vi "Day9-2.vi"() -> ()   [LabVIEW 2021]
panel:
  out "size":i32
  out "element":cluster{"x":i32, "y":i32}
  out "Array":string[](array[string])
  out "array":string[][](array[string])
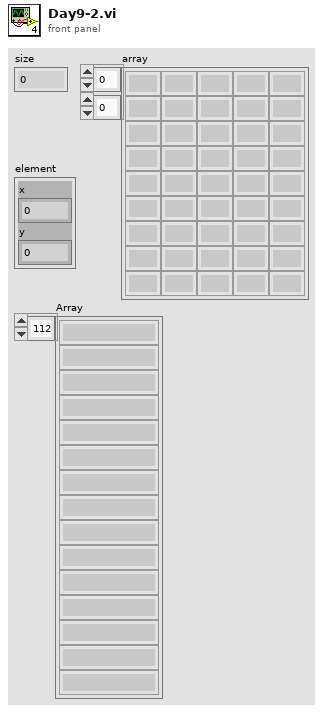
[diagram p1: front panel]
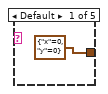
[diagram p2: hidden frame]
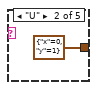
[diagram p3: hidden frame]
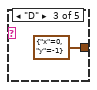
[diagram p4: hidden frame]
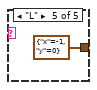
[diagram p5: hidden frame]
diagram:
  w7 = set{cluster{"x":i32, "y":i32}} {}  # Size: 0
  w11 = 10 ("dimension size")
  # "Initial starting position of Head and Tail = (0,0)"
  n1 = Spreadsheet String To Array(delimiter (Tab)=" ", format string="%s", spreadsheet string="R 2\nD 2\nR 2\nU 1\nR 2\nL 2\nD 1\nL 1\nD 2\nR 2\nU 2\nD 1\nR 2\nD 2\nU 1\nR 1\nD 1\nL 1\nU 1\nR 1\nL 1\nR 2\nU 2\nD 2\nR 2\nL 2\nU 1\nL 2\nU 2\nL 2\nR 2\nU 2\nR 1\nU 2\nL 2\nD 1\nR 1\nU 2\nD 2\nR 2\nL 2\nU 1\nD 1\nL 2\nU 2\nL 2\nU 1\nD 2\nR 1\nD 1\nR 2\nU 1\nL 2\nD 1\nU 2\nR 2\nL 1\nD 2\nU 1\nD 1\nL 1\nU 1\nR 1\nD 1\nR 1\nU 1\nD 2\nL 1\nD 1\nR 2\nD 1\nU 2\nD 2\nU 2\nL 1\nU 2\nR 2\nL 2\nD 2\nR 1\nL 2\nU 2\nL 1\nU 1\nL 1\nR 2\nL 2\nR 1\nD 1\nU 1\nL 2\nR 1\nL 1\nU 1\nD 1\nU 1\nD 1\nR 1\nL 2\nR 2\nL 1\nU 1\nD 2\nU 2\nL 2\nR 2\nU 1\nR 2\nL 2\nR 2\nL 1\nU 3\nD 1\nL 1\nD 3\nU 1\nD 2\nL 1\nR 3\nD 2\nU 3\nR 1\nD 3\nR 2\nD 1\nU 3\nL 1\nR 2\nL 3\nD 3\nU 2\nL 2\nR 3\nU 3\nD 3\nL 3\nD 2\nL 3\nR 1\nL 1\nD 1\nU 3\nD 3\nU 2\nL 3\nR 3\nU 1\nD 2\nR 2\nL 2\nD 3\nR 3\nU 1\nR 1\nL 3\nU 2\nL 2\nU 1\nR 1\nD 1\nR 3\nU 2\nD 1\nL 1\nU 1\nR 2\nL 1\nR 3\nL 1\nU 3\nL 2\nD 2\nL 2\nD 3\nL 2\nR 1\nU 2\nL 3\nD 1\nL 3\nD 1\nU 2\nL 3\nR 2\nU 1\nL 3\nD 3\nR 3\nU 2\nR 2\nD 3\nR 3\nU 2\nR 2\nL 2\nU 3\nR 1\nL 2\nD 3\nU 1\nL 1\nU 1\nL 2\nR 3\nL 3\nD 3\nR 3\nU 3\nL 1\nR 2\nD 3\nU 1\nR 2\nU 1\nD 1\nL 1\nD 2\nL 2\nD 3\nU 2\nD 1\nU 3\nD 3\nU 3\nR 3\nL 3\nU 4\nL 3\nD 1\nR 4\nU 3\nD 2\nR 1\nD 4\nL 3\nU 1\nL 1\nR 2\nD 1\nR 3\nD 3\nL 3\nD 4\nL 3\nR 4\nU 3\nR 3\nD 1\nR 3\nD 3\nR 3\nD 4\nU 4\nR 2\nD 3\nR 3\nD 2\nU 1\nR 2\nD 2\nU 2\nD 3\nL 2\nR 4\nD 4\nU 4\nR 3\nU 4\nR 1\nU 2\nR 4\nD 2\nL 4\nR 4\nU 3\nL 2\nU 2\nL 3\nR 3\nL 1\nU 4\nL 3\nU 3\nL 3\nU 1\nR 2\nU 3\nR 2\nL 3\nU 1\nD 3\nR 4\nD 1\nR 2\nL 1\nD 1\nU 2\nD 3\nR 4\nU 1\nL 3\nR 4\nU 4\nL 4\nR 2\nD 1\nU 4\nR 1\nD 3\nL 3\nD 1\nR 3\nD 2\nU 2\nL 1\nU 2\nD 3\nL 1\nU 3\nD 3\nL 3\nU 2\nL 3\nU 2\nR 1\nD 1\nR 1\nL 1\nD 2\nR 3\nD 2\nL 2\nR 3\nD 5\nR 5\nU 4\nD 5\nU 5\nD 4\nR 4\nD 2\nR 5\nL 4\nR 2\nL 2\nR 5\nU 5\nR 1\nD 2\nR 1\nL 3\nD 5\nU 3\nD 4\nR 3\nU 4\nD 1\nU 4\nL 5\nR 1\nU 4\nL 5\nU 3\nD 4\nL 2\nD 4\nU 4\nL 2\nD 1\nR 3\nD 1\nR 2\nD 4\nR 5\nL 1\nU 4\nL 4\nU 3\nL 1\nU 1\nR 4\nU 3\nL 1\nR 3\nD 5\nU 2\nR 4\nD 3\nL 2\nD 4\nR 5\nD 2\nU 3\nR 4\nD 4\nL 2\nU 4\nR 5\nL 1\nU 5\nD 1\nR 3\nL 4\nD 1\nU 3\nD 5\nR 2\nD 2\nL 5\nU 2\nD 3\nL 5\nD 5\nL 1\nR 5\nD 2\nU 3\nR 2\nL 2\nU 1\nL 5\nR 1\nL 4\nD 5\nR 5\nD 2\nU 5\nL 5\nD 1\nL 1\nD 3\nR 1\nD 2\nL 2\nR 4\nU 5\nL 2\nR 1\nU 3\nD 1\nU 1\nD 5\nR 2\nD 2\nR 3\nD 6\nU 1\nR 6\nD 4\nU 1\nR 5\nL 6\nR 2\nL 6\nU 6\nR 5\nD 2\nU 1\nD 2\nL 2\nD 5\nR 3\nU 4\nD 2\nL 1\nU 1\nD 3\nU 1\nD 1\nR 5\nU 1\nR 1\nD 3\nU 5\nL 6\nR 3\nL 6\nU 4\nD 2\nR 1\nL 6\nR 2\nD 3\nU 2\nR 2\nL 1\nD 1\nU 1\nR 4\nU 1\nR 2\nU 2\nL 2\nU 2\nD 5\nL 4\nU 6\nL 3\nD 6\nU 5\nL 6\nU 3\nR 5\nU 2\nR 4\nL 6\nD 1\nR 5\nD 4\nL 2\nR 2\nU 1\nD 2\nL 2\nU 4\nR 1\nD 2\nU 2\nR 6\nL 2\nD 5\nR 5\nL 3\nD 1\nU 1\nL 2\nD 4\nR 6\nL 5\nR 3\nU 1\nR 3\nL 1\nR 3\nU 1\nL 1\nU 4\nD 4\nU 3\nR 3\nU 1\nR 2\nD 1\nL 6\nU 2\nR 2\nD 1\nR 5\nL 2\nD 5\nL 3\nR 6\nD 2\nL 2\nD 3\nL 5\nD 7\nL 7\nD 4\nU 5\nR 7\nL 7\nD 3\nU 5\nR 6\nU 3\nL 6\nR 5\nL 4\nD 4\nR 4\nL 6\nD 6\nU 3\nD 3\nR 7\nU 1\nL 5\nU 3\nL 4\nU 3\nL 5\nD 1\nR 7\nU 3\nL 6\nD 1\nU 3\nL 2\nU 6\nL 6\nD 1\nU 1\nD 2\nL 5\nU 4\nR 5\nD 7\nU 3\nD 4\nL 1\nD 3\nR 7\nD 2\nU 4\nL 1\nD 3\nR 3\nD 6\nR 4\nU 3\nD 4\nR 6\nL 7\nU 5\nL 7\nR 3\nL 7\nD 5\nR 7\nD 4\nU 3\nR 6\nU 7\nD 2\nR 2\nL 2\nD 1\nR 3\nU 3\nD 5\nU 3\nL 3\nD 6\nL 6\nR 1\nL 5\nD 6\nU 4\nR 2\nL 2\nD 1\nU 7\nL 5\nD 3\nU 1\nL 1\nR 1\nL 6\nR 1\nD 6\nU 4\nL 7\nU 6\nR 6\nL 2\nD 5\nR 1\nD 6\nL 1\nR 3\nD 1\nU 5\nL 1\nD 3\nU 7\nD 5\nU 7\nD 7\nU 4\nR 3\nU 4\nL 8\nU 1\nR 1\nD 2\nU 5\nD 2\nL 5\nD 6\nU 4\nR 5\nL 5\nU 7\nL 3\nD 1\nL 2\nR 8\nL 1\nU 8\nL 2\nD 3\nR 6\nL 8\nD 2\nL 1\nU 4\nD 1\nR 2\nD 7\nU 5\nD 4\nU 4\nL 2\nD 6\nU 1\nD 5\nU 2\nD 2\nL 8\nD 6\nL 2\nU 1\nR 7\nD 1\nU 5\nL 6\nD 3\nL 2\nD 8\nR 6\nL 5\nU 2\nL 6\nU 4\nD 6\nL 7\nU 8\nL 5\nD 8\nR 8\nD 6\nL 3\nU 6\nL 1\nD 8\nR 7\nL 7\nR 2\nD 6\nR 1\nU 5\nL 5\nR 5\nL 3\nU 8\nL 1\nU 2\nD 5\nR 8\nU 5\nL 5\nD 2\nR 5\nU 1\nD 8\nR 3\nU 1\nR 6\nD 6\nR 5\nD 6\nL 8\nU 8\nL 8\nU 8\nL 8\nR 8\nU 8\nR 5\nL 1\nD 3\nU 1\nD 6\nU 1\nL 8\nU 3\nR 5\nL 2\nR 1\nD 2\nL 2\nU 4\nD 1\nR 1\nD 2\nR 2\nU 4\nR 3\nU 8\nD 9\nL 9\nD 5\nL 4\nD 7\nL 9\nU 4\nL 9\nD 7\nU 4\nL 3\nU 2\nR 5\nU 3\nL 1\nR 5\nL 8\nU 4\nR 6\nL 8\nU 1\nR 7\nD 6\nR 6\nU 7\nL 9\nR 7\nU 8\nR 5\nU 6\nL 4\nD 4\nL 3\nR 8\nU 6\nL 7\nR 4\nD 7\nR 3\nL 3\nD 2\nL 2\nU 5\nR 8\nL 7\nR 9\nD 8\nU 1\nL 1\nD 4\nU 6\nR 4\nL 2\nR 9\nL 9\nR 2\nD 3\nL 4\nU 6\nR 3\nD 5\nL 4\nR 8\nU 3\nR 5\nL 3\nD 7\nR 1\nD 2\nU 5\nL 7\nD 6\nR 1\nD 9\nL 9\nR 8\nU 8\nL 8\nD 7\nU 3\nL 2\nU 4\nD 8\nU 6\nR 3\nU 5\nR 7\nD 1\nR 8\nL 9\nU 7\nD 9\nL 2\nR 7\nU 1\nR 6\nD 3\nL 5\nU 10\nL 8\nR 3\nL 4\nD 9\nU 4\nL 5\nU 5\nD 10\nR 8\nU 6\nL 3\nU 4\nD 6\nL 8\nD 2\nR 8\nL 9\nU 3\nR 5\nD 1\nR 9\nD 6\nL 5\nR 10\nL 8\nR 9\nL 6\nU 8\nL 8\nU 5\nR 3\nU 6\nD 3\nL 10\nD 9\nU 5\nL 3\nU 6\nR 2\nD 7\nR 9\nL 5\nD 3\nU 3\nR 2\nD 10\nU 3\nR 2\nU 6\nL 10\nR 3\nU 3\nR 4\nL 8\nR 1\nL 6\nU 9\nL 7\nD 7\nR 6\nU 3\nR 1\nL 6\nD 5\nL 3\nU 2\nL 5\nR 9\nD 5\nR 4\nL 2\nU 5\nD 7\nL 10\nD 9\nU 7\nD 9\nR 5\nD 3\nL 1\nR 10\nL 4\nU 6\nR 7\nL 2\nR 6\nL 3\nR 3\nD 2\nL 1\nR 2\nL 7\nD 8\nR 5\nL 7\nD 8\nU 5\nL 8\nU 4\nR 8\nU 1\nD 1\nU 4\nD 6\nR 8\nU 10\nD 5\nU 5\nL 1\nD 2\nR 10\nU 10\nR 2\nL 9\nR 2\nD 3\nL 6\nR 10\nD 10\nR 9\nD 7\nU 3\nR 4\nD 9\nR 4\nD 9\nU 9\nL 8\nD 7\nR 7\nU 7\nR 7\nD 9\nL 7\nU 5\nL 10\nR 8\nL 11\nD 9\nL 5\nR 11\nL 6\nR 1\nU 2\nD 9\nL 3\nR 6\nL 6\nR 2\nL 6\nD 6\nR 2\nD 5\nL 8\nR 9\nU 6\nD 6\nL 1\nR 3\nD 2\nR 5\nD 6\nL 1\nD 10\nU 2\nR 4\nU 6\nR 11\nD 1\nR 2\nL 4\nD 9\nL 4\nU 8\nD 10\nU 4\nR 10\nD 1\nU 11\nR 2\nL 11\nD 7\nU 1\nL 7\nU 10\nD 10\nL 11\nR 1\nU 8\nR 1\nL 11\nR 3\nD 10\nR 10\nL 9\nU 7\nR 9\nL 6\nR 7\nU 5\nR 6\nU 4\nL 11\nU 7\nR 7\nL 4\nU 4\nR 2\nD 3\nR 2\nL 9\nD 4\nL 11\nR 6\nD 2\nL 9\nR 7\nD 6\nU 5\nL 8\nD 9\nR 11\nU 11\nR 6\nD 11\nL 9\nR 4\nL 6\nU 10\nR 11\nU 5\nL 6\nR 12\nD 3\nR 4\nU 12\nR 6\nD 8\nR 1\nD 2\nL 11\nR 6\nD 5\nU 10\nD 5\nR 8\nL 6\nD 5\nU 5\nR 8\nL 1\nD 10\nR 5\nU 6\nL 8\nR 4\nL 10\nD 6\nR 3\nD 9\nL 4\nR 9\nU 5\nR 2\nU 11\nR 9\nU 8\nR 7\nL 2\nD 7\nU 7\nD 8\nU 12\nR 6\nD 12\nR 5\nD 10\nU 2\nD 8\nU 6\nR 3\nU 5\nR 5\nL 11\nD 10\nR 3\nU 11\nD 8\nR 7\nL 3\nU 9\nR 4\nL 2\nD 4\nR 8\nD 9\nR 2\nD 3\nU 6\nL 5\nD 4\nL 2\nR 9\nU 5\nD 1\nU 9\nR 9\nU 11\nL 12\nR 10\nD 5\nU 1\nR 9\nU 4\nD 8\nR 1\nD 5\nR 7\nU 11\nL 6\nU 1\nR 12\nD 1\nR 7\nU 12\nD 9\nR 12\nL 1\nU 3\nD 6\nR 11\nL 6\nU 8\nD 11\nR 7\nU 5\nD 4\nU 1\nL 11\nD 1\nU 5\nR 13\nL 9\nU 4\nD 4\nR 10\nU 4\nD 7\nL 4\nD 10\nR 6\nD 5\nR 9\nL 10\nD 2\nU 11\nD 8\nU 1\nR 8\nU 5\nR 8\nD 10\nL 10\nD 7\nR 5\nU 6\nD 7\nU 9\nR 8\nD 4\nR 2\nD 1\nL 1\nU 2\nR 10\nD 2\nU 13\nL 9\nU 13\nL 12\nU 12\nD 6\nL 1\nR 4\nL 7\nR 4\nL 2\nU 8\nR 7\nD 10\nU 2\nL 8\nD 5\nR 9\nD 9\nR 2\nL 3\nU 2\nD 11\nU 5\nD 12\nR 3\nU 10\nD 2\nR 1\nD 13\nU 7\nL 7\nR 1\nU 1\nR 1\nU 6\nD 12\nR 7\nL 7\nR 9\nU 10\nR 13\nD 3\nR 12\nU 1\nL 6\nR 9\nU 10\nL 1\nU 13\nR 2\nD 8\nU 12\nD 10\nL 7\nU 6\nD 9\nL 11\nD 8\nU 4\nR 1\nD 11\nL 8\nU 1\nD 4\nR 7\nU 7\nR 5\nL 1\nR 14\nL 8\nD 10\nR 13\nU 13\nR 9\nL 13\nU 2\nD 7\nR 11\nD 2\nL 9\nD 11\nL 2\nU 12\nD 11\nR 12\nD 3\nR 6\nL 11\nR 7\nD 3\nU 6\nD 9\nL 10\nR 13\nD 7\nU 14\nL 10\nR 11\nD 12\nR 12\nU 13\nR 4\nL 14\nU 5\nL 4\nU 10\nL 3\nU 13\nR 9\nD 7\nU 8\nR 5\nL 14\nU 5\nR 6\nD 13\nL 13\nU 9\nR 13\nD 1\nL 8\nR 9\nU 8\nL 7\nU 4\nD 4\nR 4\nL 5\nU 11\nR 14\nL 2\nU 1\nD 14\nR 13\nD 3\nL 13\nD 2\nU 9\nD 14\nU 1\nR 1\nD 12\nL 6\nR 4\nU 4\nL 11\nU 14\nD 13\nR 12\nL 7\nU 13\nR 4\nU 14\nL 14\nR 11\nL 8\nD 3\nU 4\nR 1\nU 5\nD 12\nL 5\nU 14\nD 6\nR 6\nU 4\nL 1\nD 11\nU 9\nR 5\nU 13\nD 7\nL 5\nD 3\nL 8\nU 7\nD 4\nL 13\nR 1\nD 11\nL 7\nU 6\nD 9\nR 10\nD 6\nR 9\nL 2\nD 6\nU 12\nL 10\nD 3\nU 6\nL 4\nR 4\nU 12\nD 13\nR 9\nL 1\nR 5\nU 14\nR 14\nD 7\nU 10\nR 3\nL 4\nU 6\nL 13\nU 14\nR 10\nL 7\nD 12\nU 5\nL 11\nD 7\nU 9\nD 4\nL 1\nR 11\nD 9\nL 5\nD 15\nR 4\nU 12\nL 1\nU 8\nL 15\nD 15\nL 3\nR 11\nL 9\nR 1\nU 12\nD 9\nR 7\nD 6\nU 2\nL 12\nU 13\nR 11\nL 15\nD 4\nL 8\nU 6\nL 7\nR 2\nU 7\nD 2\nU 13\nD 10\nL 13\nU 1\nD 6\nL 11\nR 14\nL 5\nU 2\nR 11\nD 10\nL 4\nR 14\nU 13\nD 9\nU 2\nD 4\nR 14\nL 4\nR 4\nL 4\nU 6\nD 11\nL 10\nU 9\nL 3\nU 12\nL 8\nU 9\nD 4\nU 4\nL 10\nU 1\nD 8\nU 15\nD 3\nU 12\nR 3\nD 8\nU 1\nR 10\nL 1\nU 5\nD 1\nL 1\nR 3\nU 1\nR 8\nU 10\nR 1\nU 11\nR 15\nD 16\nU 13\nD 7\nU 7\nD 14\nR 9\nL 13\nR 12\nU 2\nR 11\nL 11\nR 3\nD 11\nU 11\nR 2\nD 3\nU 6\nL 14\nR 6\nL 6\nU 3\nR 3\nD 1\nU 5\nL 3\nR 4\nD 9\nU 15\nR 2\nU 5\nD 5\nR 14\nU 6\nR 1\nD 4\nU 2\nD 3\nR 8\nL 4\nD 2\nU 12\nD 2\nU 7\nL 14\nU 1\nR 10\nL 4\nD 12\nL 9\nD 16\nU 2\nR 7\nD 16\nU 9\nD 13\nU 7\nL 14\nD 5\nR 12\nU 13\nR 13\nU 2\nL 11\nD 9\nU 2\nR 8\nU 5\nR 7\nU 9\nL 11\nD 16\nU 10\nR 5\nD 7\nL 6\nD 8\nU 4\nR 3\nD 5\nL 5\nU 11\nR 4\nD 12\nR 12\nL 10\nR 15\nU 9\nD 12\nL 11\nU 6\nD 11\nU 12\nL 6\nR 3\nU 12\nD 5\nL 1\nR 12\nU 14\nL 1\nD 2\nL 4\nD 7\nL 12\nU 10\nL 12\nU 4\nD 14\nR 13\nU 9\nL 2\nU 6\nL 1\nU 9\nD 16\nL 2\nR 16\nD 5\nL 7\nU 13\nL 15\nR 1\nD 8\nR 15\nD 5\nR 12\nL 5\nR 11\nU 17\nD 13\nU 13\nL 4\nD 8\nL 1\nD 7\nR 11\nU 7\nR 11\nL 9\nD 3\nL 2\nU 4\nD 16\nL 10\nU 11\nR 5\nU 4\nR 6\nL 11\nR 17\nU 13\nR 12\nD 11\nL 17\nU 15\nD 4\nR 9\nU 9\nL 10\nD 5\nR 14\nU 10\nR 5\nU 15\nL 12\nD 14\nR 14\nL 11\nR 5\nU 7\nD 1\nR 4\nD 14\nU 3\nR 6\nD 5\nR 1\nD 12\nL 14\nD 6\nL 15\nU 16\nD 10\nR 12\nD 9\nU 1\nD 1\nL 4\nD 6\nU 16\nR 11\nL 11\nR 3\nL 2\nU 12\nR 9\nD 16\nR 12\nL 14\nU 6\nL 7\nD 5\nU 4\nR 13\nL 8\nD 16\nU 5\nD 5\nU 6\nR 14\nL 6\nD 7\nU 3\nL 15\nR 14\nL 17\nR 17\nU 16\nL 4\nR 3\nU 1\nD 15\nL 12\nD 11\nL 18\nD 18\nU 10\nD 4\nU 1\nR 11\nU 18\nD 12\nR 11\nU 13\nD 14\nR 17\nD 18\nU 13\nR 8\nU 4\nR 9\nD 18\nL 6\nR 7\nL 14\nU 10\nL 10\nU 16\nD 15\nL 15\nD 3\nL 2\nD 7\nR 3\nD 7\nU 11\nL 6\nR 8\nL 3\nU 3\nR 8\nD 8\nU 10\nL 15\nD 1\nU 16\nR 1\nL 13\nR 7\nU 10\nL 12\nR 8\nD 3\nL 14\nD 12\nR 12\nD 3\nL 2\nD 15\nR 3\nL 14\nD 4\nR 5\nL 13\nD 9\nU 2\nL 5\nR 13\nD 4\nL 14\nR 14\nD 16\nR 1\nU 11\nR 6\nL 7\nU 16\nL 15\nD 6\nU 7\nR 16\nD 2\nL 15\nD 18\nU 3\nD 1\nR 7\nD 1\nL 4\nD 16\nU 12\nL 12\nR 7\nU 5\nL 5\nU 13\nR 13\nU 7\nL 9\nR 9\nU 8\nD 6\nL 3\nU 4\nR 12\nL 12\nD 16\nU 12\nL 4\nR 11\nU 9\nD 13\nR 15\nL 3\nD 17\nR 6\nD 13\nR 6\nD 5\nL 19\nU 10\nD 3\nL 2\nU 13\nR 2\nD 3\nL 3\nU 3\nR 1\nU 12\nL 2\nD 19\nL 17\nR 10\nD 11\nU 8\nR 10\nL 15\nR 4\nD 9\nU 4\nD 11\nU 4\nD 3\nL 5\nD 15\nU 1\nL 19\nD 16\nR 11\nU 12\nD 16\nL 4\nR 13\nU 2\nL 19\nU 9\nR 5\nD 7\nR 19\nL 9\nU 2\nD 2\nR 3\nU 10\nL 13\nD 16\nL 2\nD 5\nL 8\nR 9\nL 18\nR 9\nU 13\nD 7\nR 14\nU 8\nR 18\nL 18\nU 8\nL 13\nR 9\nU 5\nL 16\nU 4\nD 4\nR 10\nU 13\nR 2\nL 6\nR 18\nD 3\nL 11\nR 12\nL 2\nR 12\nD 7\nU 12\nR 13\nU 14\nD 1\nR 8\nL 13\nU 5\nL 9\nU 19\nD 14\nL 4\nU 8\nD 8\nU 1\nD 16\nU 4\nD 8\nU 20", array type (2D Dbl)=string[][] []) -> (array=w15:string[][])
  "array" <- w15
  n2 = Initialize Array(cluster{"x":i32, "y":i32} {"x"=0, "y"=0} ("Head"), w11) -> (w13:cluster{"x":i32, "y":i32}[])
  n3 = for {
    tunnel: w15 -> [w23] mode=indexing
    tunnel: [w19] -> w10 mode=concatenating
    n4 = Index Array(array=w23) -> (element #1=w20:string, element #2=w22:string)  [unwired: 2 in]
    n5 = Decimal String To Number(string=w22) -> (number=w21:i32)  [unwired: 2 in, 1 out]
    n6 = Initialize Array(w20, w21) -> (w19:string[])
  }
  "Array" <- w10
  n7 = for {
    tunnel: w10 -> [w32] mode=indexing
    shift-right: [w24] -> _
    shift-left: w13 -> [w31]
    tunnel: [w24] -> w12 mode=indexing
    n8 = in-place {
      in-place-border: w32 -> [w42]
      n9 = in-place-array #1(w31, 0) -> (w40:cluster{"x":i32, "y":i32})
      n10 = case shown="\"R\"" w42 {
        tunnel: [cluster{"x":i32, "y":i32} {"x"=0, "y"=0} ("Tail") cluster{"x":i32, "y":i32} {"x"=0, "y"=1} ("Tail") cluster{"x":i32, "y":i32} {"x"=0, "y"=-1} ("Tail") cluster{"x":i32, "y":i32} {"x"=1, "y"=0} ("Tail") cluster{"x":i32, "y":i32} {"x"=-1, "y"=0} ("Tail")] -> w41
        frame Default {
        }
        frame "U" {
        }
        frame "D" {
        }
        frame "R" {
        }
        frame "L" {
        }
      }
      n11 = Add(x=w41, y=w40) -> (x+y=w39:cluster{"x":i32, "y":i32})
      n12 = in-place-array #1(w39) -> (w30:cluster{"x":i32, "y":i32}[])  [unwired: 1 out]
    }
    n13 = Index Array(array=w30) -> (element=w26:cluster{"x":i32, "y":i32})  [unwired: 1 in]
    n14 = Array Size(array=w30) -> (size(s)=w29:i32)
    n15 = Decrement(x=w29) -> (x-1=w28:i32)
    n16 = for {
      N: w28 -> [_]
      shift-right: [w33] -> _
      shift-left: w26 -> [w34]
      tunnel: w30 -> [w37]
      tunnel: [w33] -> w27 mode=indexing
      i -> [w38]
      n17 = Increment(x=w38) -> (x+1=w36:i32)
      n18 = Index Array(array=w37, index=w36) -> (element=w35:cluster{"x":i32, "y":i32})
      n19 = call "Compute Tail Movement and New Position.vi"("Tail in"=w35, "Head"=w34) -> ("Tail out"=w33:cluster{"x":i32, "y":i32})  [unwired: 9 in]
    }
    n20 = Build Array (concatenate)(w26, w27) -> (w24:cluster{"x":i32, "y":i32}[])
  }
  n21 = Array Size(array=w10) -> (size(s)=w9:i32)
  n22 = Decrement(x=w11) -> (x-1=w4:i32)
  n23 = Build Array (concatenate)(w13, w12) -> (w3:cluster{"x":i32, "y":i32}[][])
  n24 = Index Array(array=w3, index (row)=w9, index (col)=w4) -> (element=→"element":cluster{"x":i32, "y":i32})
  n25 = Index Array(array=w3, index (col)=w4) -> (element=w2:cluster{"x":i32, "y":i32}[])  [unwired: 1 in]
  n26 = for {
    tunnel: w2 -> [w49] mode=indexing
    shift-right: [w48] -> w6
    shift-left: w7 -> [w50]
    n27 = Insert Into Set(10:w49, 11:w50) -> (3:w48:set{cluster{"x":i32, "y":i32}})  [unwired: 1 out]
  }
  n28 = Collection Size(1:w6) -> (0:→"size":i32)
